vi "JPL Drivetrain Ramps.vi"(6 "Enable Ramps":bool, 8 "Right Joystick Input":dbl(slide) scale=-10.0..10.0, 10 "Delay Time (s)":dbl, 11 "Left Joystick Input":dbl(slide) scale=-10.0..10.0) -> (0 "Right Track Out":dbl, 3 "Left Track Out":dbl)   [LabVIEW 2015]
panel:
  in  "Enable Curves":bool
  out "Waveform Chart 2":cluster{"Slide":dbl, "Slide":dbl}(graph)
  out "Waveform Chart":cluster{"Slide":dbl, "Slide":dbl}(graph)
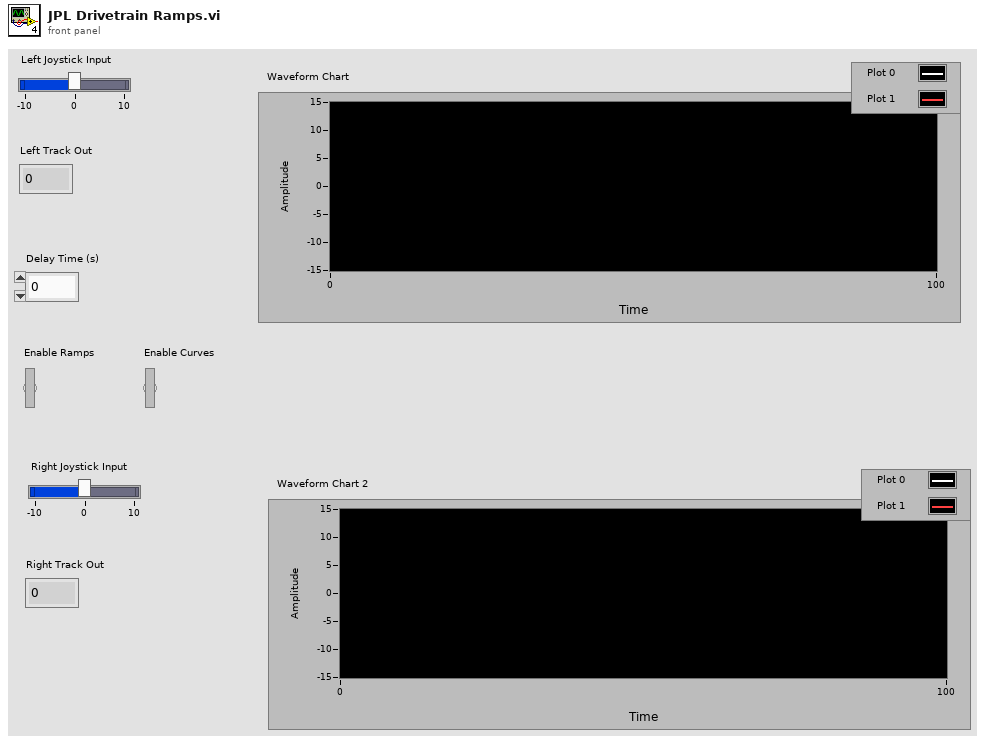
[diagram p1: front panel]
types:
  T1 = cluster{"Right Joystick Input":dbl, "Right Joystick Input":dbl}
  T2 = cluster{"Left Joystick Input":dbl, "Left Joystick Input":dbl}
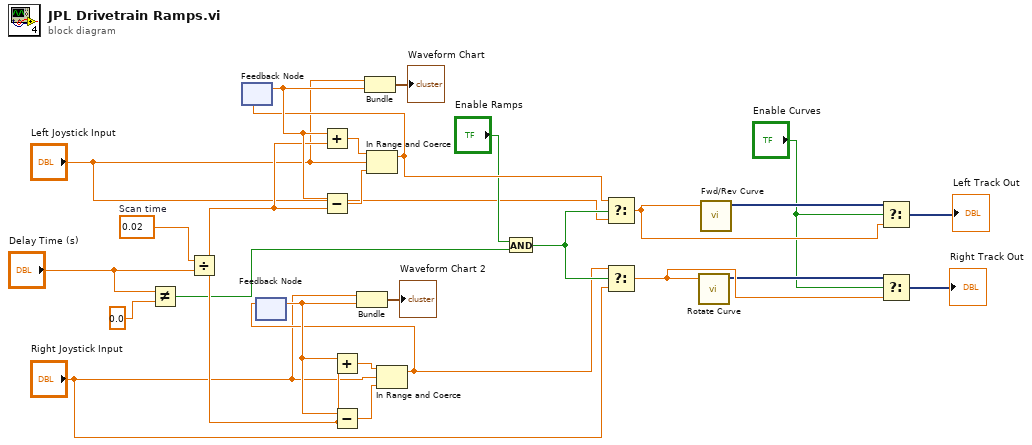
[diagram p0: block diagram]
diagram:
  w17 = 0.02  # Scan time
  n1 = Not Equal?(x="Delay Time (s)", y=0.0) -> (x != y?=w11:bool)
  n2 = Divide(x=w17, y="Delay Time (s)") -> (x/y=w16:dbl)
  n3 = feedback #1() -> (w23:dbl)  [unwired: 1 in]
  n4 = feedback #2() -> (w19:dbl)  [unwired: 1 in]
  n5 = Add(x=w23, y=w16) -> (x+y=w26:dbl)
  n6 = Subtract(x=w23, y=w16) -> (x-y=w25:dbl)
  n7 = Add(x=w19, y=w16) -> (x+y=w22:dbl)
  n8 = Subtract(x=w19, y=w16) -> (x-y=w21:dbl)
  n9 = Bundle("Right Joystick Input"="Right Joystick Input", "Right Joystick Input"=w19) -> (→"Waveform Chart 2":T1)  [unwired: 1 in]
  n10 = Bundle("Left Joystick Input"="Left Joystick Input", "Left Joystick Input"=w23) -> (→"Waveform Chart":T2)  [unwired: 1 in]
  n11 = In Range and Coerce(upper limit=w26, x="Left Joystick Input", lower limit=w25) -> (coerced(x)=w18:dbl)  [unwired: 1 out]
  n12 = feedback-in #1(w18) -> ()
  n13 = In Range and Coerce(upper limit=w22, x="Right Joystick Input", lower limit=w21) -> (coerced(x)=w10:dbl)  [unwired: 1 out]
  n14 = feedback-in #2(w10) -> ()
  n15 = And(x="Enable Ramps", y=w11) -> (x .and. y?=w15:bool)
  n16 = Select(t=w18, s=w15, f="Left Joystick Input") -> (s? t:f=w7:dbl)
  n17 = Select(t=w10, s=w15, f="Right Joystick Input") -> (s? t:f=w6:dbl)
  n18 = call "Rotate Curve"("Signals"=w6) -> ("Scaled Signals"=w5:dynamicdata)  [unwired: 9 in, 1 out]
  n19 = call "Fwd/Rev Curve"("Signals"=w7) -> ("Scaled Signals"=w4:dynamicdata)  [unwired: 9 in, 1 out]
  n20 = Select(t=w4, s="Enable Curves", f=w7) -> (s? t:f=→"Left Track Out":dynamicdata)
  n21 = Select(t=w5, s="Enable Curves", f=w6) -> (s? t:f=→"Right Track Out":dynamicdata)
